vi "Intake3 Controller.vi"(8 "error in":errorcluster) -> ()   [LabVIEW 2020]
doc: "This VI executes continuously carrying out the current operation and responding to updates or new operations. It will often contain the timing or control code that is difficult to place directly in TeleOp. This VI generally opens all sensors and motors and isolates the rest of the robot code from knowing how the operations are carried out."
uses:
  <vilib>/Rock Robotics/WPI/Framework/Completion Status.ctl
  Intake3 Setpoints.ctl
  Intake3 Operations.ctl
  <vilib>/Rock Robotics/Network Tables/NT Write Number.vi
panel:
  in  "Interactive Values":T1
  out "Current\nCmd":string
  in  "Buttons":cluster{"Execute Cmd":bool, "Abort Cmd":bool}
  out "Command Timing":cluster{"Start Time (ms)":u32, "Iterations":i32}
  out "Status":T3
  # "Tip: It may be helpful to observe inputs and sensor values.\nYou may also want to display tuning or debugging controls."
  # "Interactive Command: You may fill in the settings for a command\nand schedule it with the Execute button. You can observe and abort\nany command while fine tuning the code for the controller."
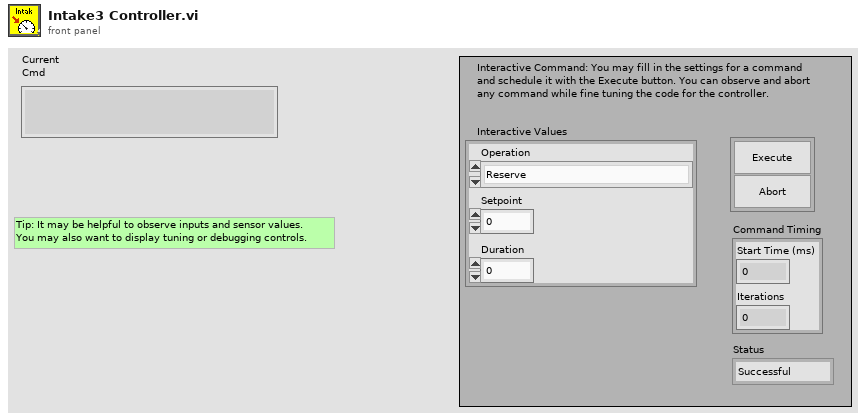
[diagram p1: front panel]
types:
  T1 = typedef "Intake3 Setpoints.ctl" = cluster{"Operation":T2, "Setpoint":dbl, "Duration":dbl}
  T2 = typedef "Intake3 Operations.ctl" = enum16{"Reserve", "Read Current", "Immediate", "for Duration", "Stop"}
  T3 = typedef "Completion Status.ctl" = enum16{"Successful", "Aborted", "Incomplete"}
  T4 = typedef "WPI_MotorControlDeviceRef.ctl" = cluster{"DeviceStatus":errorcluster, "Type":T5, "PWM":cluster{"PWM Channel":T6, "DeadBand":T7}, "CAN":cluster{"Device Number":u8, "SetOutput VI Ref":variant, "GetOutput VI Ref":variant, "Enable VI Ref":variant, "Disable VI Ref":variant, "Data":variant}, "Invert":bool, "DIO PWM":cluster{"PWM \"Enable\" Channel":T6, "DIOChannel":T8, "PWM Rate":dbl}}
  T5 = typedef "WPI_MotorControlType.ctl" = enum16{"PWM", "CAN", "DIO PWM"}
  T6 = typedef "FPGA_DIOPWMChannel.ctl" = enum8{"PWM 0", "PWM 1", "PWM 2", "PWM 3", "PWM 4", "PWM 5", "PWM 6", "PWM 7", "PWM 8", "PWM 9", "PWM MXP 0", "PWM MXP 1", "PWM MXP 2", "PWM MXP 3", "PWM MXP 4", "PWM MXP 5", "PWM MXP 6", "PWM MXP 7", "PWM MXP 8", "PWM MXP 9", "Invalid"}
  T7 = typedef "WPI_PWMDeadband.ctl" = cluster{"Name":string, "maxPositivePwm":i32, "minPositivePwm":i32, "centerPwm":i32, "maxNegativePwm":i32, "minNegativePwm":i32, "angularRange":u16}
  T8 = typedef "FPGA_DIOChannel.ctl" = enum8{"DIO 0", "DIO 1", "DIO 2", "DIO 3", "DIO 4", "DIO 5", "DIO 6", "DIO 7", "DIO 8", "DIO 9", "DIO MXP 0", "DIO MXP 1", "DIO MXP 2", "DIO MXP 3", "DIO MXP 4", "DIO MXP 5", "DIO MXP 6", "DIO MXP 7", "DIO MXP 8", "DIO MXP 9", "DIO MXP 10", "DIO MXP 11", "DIO MXP 12", "DIO MXP 13", "DIO MXP 14", "DIO MXP 15", "SPI Port CS1", "SPI Port CS2", "SPI Port CS3", "SPI Port MISO", "SPI Port MOSI", "Invalid"}
  T9 = typedef "Command Status Info.ctl" = cluster{"Name":string, "Status":T3, "notifier out":T10}
  T10 = typedef "Completion Notifier.ctl" = refnum<notifier>
  T11 = cluster{"Current Command":T1, "Command Timing":cluster{"Start Time (ms)":u32, "Iterations":i32}, "Command Arguments":cluster{"Command Info":T9, "Description":string, "Default Command":T1, "queue out":refnum<queue>, "Subsystem Name":string}}
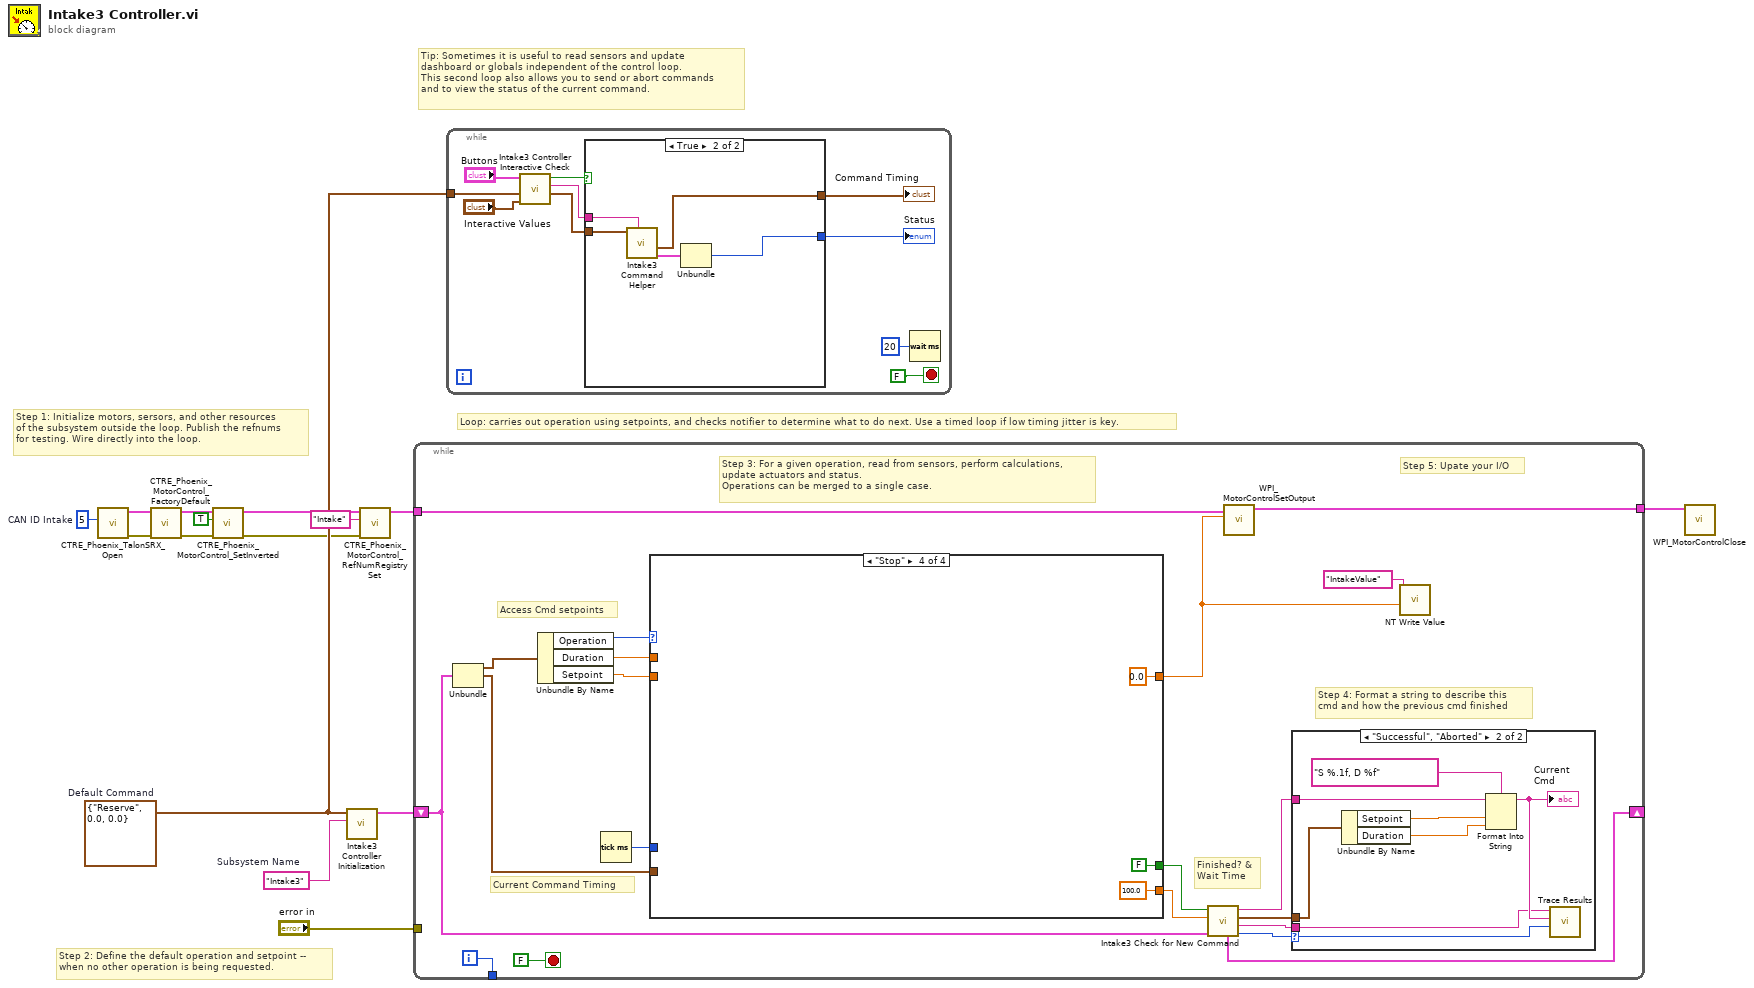
[diagram p0: block diagram]
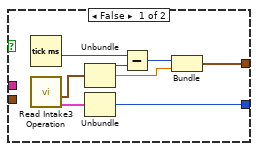
[diagram p2: hidden frame]
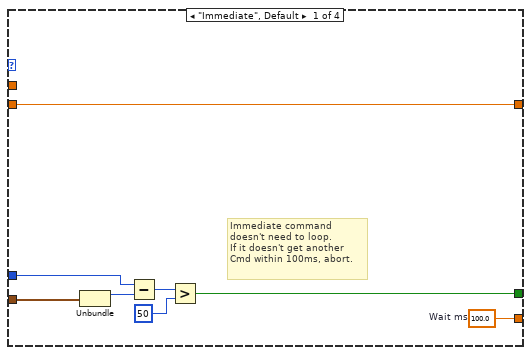
[diagram p4: hidden frame]
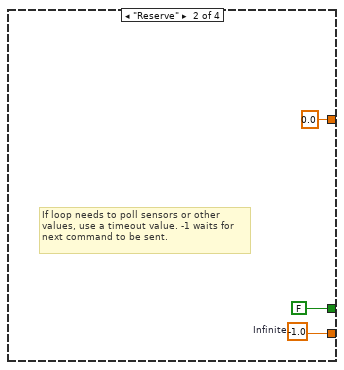
[diagram p5: hidden frame]
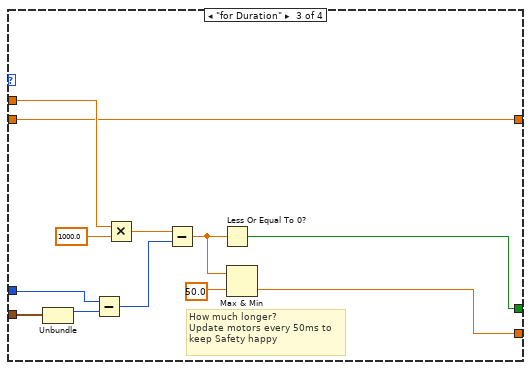
[diagram p6: hidden frame]
diagram:
  w3 = u8 5  # CAN ID Intake
  w12 = T1 {"Operation"=enum."Reserve", "Setpoint"=0.0, "Duration"=0.0}  # Default Command
  w13 = "Intake3"  # Subsystem Name
  # "Tip: Sometimes it is useful to read sensors and update\ndashboard or globals independent of the control loop.\nThis second loop also allows you to send or abort commands\nand to view the status of the current command."
  # "Step 2: Define the default operation and setpoint --\nwhen no other operation is being requested."
  # "Step 1: Initialize motors, sersors, and other resources\nof the subsystem outside the loop. Publish the refnums\nfor testing. Wire directly into the loop."
  # "Loop: carries out operation using setpoints, and checks notifier to determine what to do next. Use a timed loop if low timing jitter is key."
  n1 = call <vilib>:"CTRE_Phoenix_TalonSRX_Open.vi"("Device Number"=w3) -> ("error out"=w11:errorcluster, "PhoenixMotorControlDevRef"=w10:T4)  [unwired: 9 in]
  n2 = call <vilib>:"CTRE_Phoenix_MotorControl_FactoryDefault.vi"("error in"=w11, "PhoenixMotorControlDevRef"=w10) -> ("error out"=w9:errorcluster, "PhoenixMotorControlDevRef"=w8:T4)  [unwired: 8 in]
  n3 = call <vilib>:"CTRE_Phoenix_MotorControl_SetInverted.vi"("error in (no error)"=w9, "Invert?"=TRUE, "PhoenixMotorControlDevRef"=w8) -> ("error out"=w7:errorcluster, "PhoenixMotorControlDevRef"=w6:T4)  [unwired: 7 in]
  n4 = call "Intake3 Controller Initialization.vi"("Subsystem Name"=w13, "Default Command"=w12) -> ("Current Command"=w14:T11)  [unwired: 9 in]
  n5 = call <vilib>:"CTRE_Phoenix_MotorControl_RefNumRegistrySet.vi"("error in (no error)"=w7, "refnum name"="Intake", "PhoenixMotorControlDevRef"=w6) -> ("PhoenixMotorControlDevRef"=w2:T4)  [unwired: 7 in, 1 out]
  n6 = while {
    shift-right: [w27] -> _
    shift-left: w14 -> [w20]
    tunnel: [w34] -> _
    tunnel: "error in" -> [_]
    tunnel: w2 -> [w19]
    tunnel: [w18] -> w1
    i -> [w34]
    stop <- FALSE stop-if-true
    # "Step 5: Upate your I/O"
    # "Step 4: Format a string to describe this\ncmd and how the previous cmd finished"
    # "Current Command Timing"
    # "Access Cmd setpoints"
    # "Finished? &\nWait Time"
    # "Step 3: For a given operation, read from sensors, perform calculations,\nupdate actuators and status.\nOperations can be merged to a single case."
    n7 = Unbundle(w20) -> ("Current Command"=w33:T1, "Command Timing"=w29:cluster{"Start Time (ms)":u32, "Iterations":i32})  [unwired: 1 out]
    n8 = Unbundle By Name(w33) -> ("Operation"=w32:T2, "Duration"=w31:dbl, "Setpoint"=w28:dbl)
    n9 = Tick Count (ms)() -> (millisecond timer value=w30:u32)
    n10 = case shown="\"Stop\"" w32 {
      tunnel: [w51 w54 w56 100.0 ("Infinite")] -> w25
      tunnel: [w45 FALSE ("ignore previous (F)") w57 FALSE ("ignore previous (F)")] -> w26
      tunnel: w29 -> [w47 _ w59 _]
      tunnel: w31 -> [_ _ w58 _]
      tunnel: w30 -> [w46 _ w60 _]
      tunnel: w28 -> [w44 _ w55 _]
      tunnel: [w44 0.0 ("Setpoint") w55 0.0 ("Setpoint")] -> w17
      frame "Immediate", Default {
        w51 = 100.0  # Wait ms
        # "Immediate command\ndoesn't need to loop.\nIf it doesn't get another\nCmd within 100ms, abort."
        n11 = Unbundle(w47) -> ("Start Time (ms)"=w50:u32)  [unwired: 1 out]
        n12 = Subtract(x=w46, y=w50) -> (x-y=w49:u32)
        n13 = Greater?(x=w49, y=u8 50 ("Left Motor")) -> (0:w45:bool)
      }
      frame "Reserve" {
        w54 = -1.0  # Infinite
        # "If loop needs to poll sensors or other\nvalues, use a timeout value. -1 waits for\nnext command to be sent."
      }
      frame "for Duration" {
        # "How much longer?\nUpdate motors every 50ms to\nkeep Safety happy"
        n14 = Unbundle(w59) -> ("Start Time (ms)"=w63:u32)  [unwired: 1 out]
        n15 = Subtract(x=w60, y=w63) -> (x-y=w66:u32)
        n16 = Multiply(x=w58, y=1000.0) -> (x*y=w65:dbl)
        n17 = Subtract(x=w65, y=w66) -> (x-y=w62:dbl)
        n18 = Less Or Equal To 0?(x=w62) -> (x <= 0?=w57:bool)
        n19 = Max & Min(x=w62, y=50.0) -> (min(x,y)=w56:dbl)  [unwired: 1 out]
      }
      frame "Stop" {
      }
    }
    n20 = call "Intake3 Check for New Command.vi"("Current Command"=w20, "Wait time (ms)"=w25, "Finished?"=w26) -> ("Completion"=w21:T3, "Subsystem Name"=w22:string, "Current Command"=w23:T1, "Initial Trace String"=w24:string, "NextCommand"=w27:T11)  [unwired: 4 in]
    n21 = call <vilib>:"WPI_MotorControlSetOutput.vi"("Output"=w17, "MotorControlDevRef"=w19) -> ("MotorControlDevRef"=w18:T4)  [unwired: 7 in, 2 out]
    n22 = case shown="\"Successful\", \"Aborted\"" w21 {
      selector: w21 -> [_ w43]
      tunnel: w24 -> [_ w39]
      tunnel: w23 -> [_ w40]
      tunnel: w22 -> [_ w36]
      frame "Incomplete", Default {
        # "Continuing current command"
      }
      frame "Successful", "Aborted" {
        # "Report and setup for next command"
        n23 = Unbundle By Name(w40) -> ("Setpoint"=w42:dbl, "Duration"=w37:dbl)
        n24 = Format Into String(format string="S %.1f, D %f", initial string=w39, w42, w37) -> (resulting string=w38:string)  [unwired: 1 in, 1 out]
        "Current\nCmd" <- w38
        n25 = call <vilib>:"Trace Results.vi"("Status of previous command"=w43, "Description"=w38, "Subsystem"=w36) -> ()  [unwired: 9 in]
      }
    }
    n26 = call-poly <vilib>:"NT Write Value.vi"("Numeric"=w17, "Name"="IntakeValue") -> ()  [unwired: 9 in, 1 out]
  }
  n27 = while {
    tunnel: w12 -> [w76]
    stop <- FALSE stop-if-true
    n28 = call "Intake3 Controller Interactive Check.vi"("Interactive Command in"="Interactive Values", "Default Command"=w76, "Buttons"="Buttons") -> ("Interactive Command out"=w73:T1, "Trace String"=w74:string, "Schedule"=w75:bool)  [unwired: 6 in]
    n29 = case shown="True" w75 {
      tunnel: [w87 w92] -> w72
      tunnel: w73 -> [_ w90]
      tunnel: [w83 w88] -> w71
      tunnel: w74 -> [_ w91]
      frame False {
        n30 = Tick Count (ms)() -> (millisecond timer value=w82:u32)
        n31 = call "Read Intake3 Operation.vi"() -> ("Command Info"=w80:T9, "SubSystem Data"=w81:T1)  [unwired: 9 in, 1 out]
        n32 = Unbundle(w81) -> ("Operation"=w86:T2, "Setpoint"=w84:dbl)  [unwired: 1 out]
        n33 = Unbundle(w80) -> ("Status"=w87:T3)  [unwired: 2 out]
        n34 = Subtract(x=w82, y=w86) -> (x-y=w85:u32)
        n35 = Bundle(w85, "Setpoint"=w84) -> (w83:cluster{u32, "Setpoint":dbl})  [unwired: 1 in]
      }
      frame True {
        n36 = call "Intake3 Command Helper.vi"("Description"=w91, "SubSystem Data"=w90) -> ("Command Info Out"=w89:T9, "Command Timing"=w88:cluster{"Start Time (ms)":u32, "Iterations":i32})  [unwired: 7 in, 1 out]
        n37 = Unbundle(w89) -> ("Status"=w92:T3)  [unwired: 2 out]
      }
    }
    "Status" <- w72
    "Command Timing" <- w71
    n38 = Wait (ms)(milliseconds to wait=u32 20) -> ()  [unwired: 1 out]
  }
  n39 = call <vilib>:"WPI_MotorControlClose.vi"("MotorControlDevRef"=w1) -> ()  [unwired: 10 in, 1 out]
